vi "Read Support Script.vi"(6 "Error In":errorcluster, 8 "Support Script":path, 9 "Data In":T1={"Message"="", "Homed?"=FALSE, "NextState"=enum."Timeout", "G.Load"=0.0, "G.Position"=0.0, "Load#"=0, "[G.Loads]"=[], "[TotalLoads]"=[], "[Errors]"=[], "ZeroWait"=0, "Results"=[], "DwellWait"=FALSE, "Test Result"=FALSE, "[CondyleLoads]"=[], "[Max]"=[], "[Min]"=[], "Valid String?"=FALSE, "ScanTime"=timestamp(0 s since 1904-01-01), "ScannedString"="", "LabelDevID"=0, "MfgDate"=timestamp(0 s since 1904-01-01), "[EEPROM Cmds]"=[], "[CalData]"=[], "[A/Ds]"=[], "[A/Dmax]"=[], "[A/Dmin]"=[], "BattMax"=0.0, "BattMin"=0.0, "DwellTime"=2000, "PendingDeviceType"="", "Zero G.load"=0.0, "GAINC Value"="", "Programming Step"=enum."Load EEPROM", "Front Panel Program?"=FALSE, "Final Program?"=FALSE, "PCB Score"=100, "AssyScore"=100, "Pass/Fail #"="", "Result String"="", "Programming Mode"=enum."Initial Program", "Angle Test Step"=enum."Initialize", "Accel Values"=[], "Shutdown Counter"=0, "V1"=0, "V2"=0, "V3"=0, "V4"=0, "EEPROM Data"=[], "Counter"=0, "Page#"=0, "Timer"=timestamp(0 s since 1904-01-01), "Use Mark10?"=FALSE, "Eng-Result#"=0, "DUT Serial #"=0, "Scroll Message?"=FALSE, "Clear Message"=FALSE, "Batt Test Step "=enum."Initialize", "RXTX Window Found?"=FALSE, "Shutdown First Call?"=FALSE, "A2 Delay (msec)"=500, "Support Script"={"Script #"="", "Script Revision"="", "[OEMs]"=[], "[[DeviceTypes]]"=[], "[[DeviceTypesVals]]"=[], "[[List of Errors]]"=[], "Default GAINC"="", "[[ASICtrims]]"=[], "ID For Echo"="", "Condyle A CalFactor"=100, "Condyle B CalFactor"=100, "[OEMs Prefix]"=[], "Packet ID 18"="", "[[Force Table Load Test]]"=[], "[[Force Table AccurTest]]"=[]}, "Serial Table"={"Serial File Path"=path "", "[[Serial Lookup Table]]"=[], "Serial Device Info"=[], "Valid Serial?"=FALSE}, "Target Information"={"Target Brand"="", "Target DeviceType"="", "Target Serial#"=100, "Target Lot#"=0, "Target DevID"=0, "Target Channel"=5}, "Operator"="", "COM Port"="", "Config Path"=path "", "Tx Array"=[], "DUT Parameters"={"Channel"=0, "DeviceID"=0, "Script Rev"=0, "Month"=0, "Day"=0, "Year"=0, "Lot#"=0, "V1"=0, "V2"=0, "V3"=0, "V4"=0, "MFG"=0, "Cal FactorA 10"=0, "Cal FactorB 10  "=0, "Cal FactorA 16"=0, "Cal FactorB 16"=0, "ASICtrim"=[], "TmpChan"=0, "GAINC"="", "Brand"="", "Device"="", "Serial #"=0, "Batt310"=0, "Batt 280"=0}, "FTS Main?"=FALSE, "Loading"={"[Forces]"=[], "[Dwell]"=[], "Loading Step"=enum."Initialize Test"}, "Software Version"="", "Correction Factor"="", "Second Load Test"=FALSE, "Acc Loads"=[], "Mark10 Config"={"H2S%"=[80.0, 85.0, 90.0, 95.0, 100.0], "H2S Speed"=[12.0, 8.0, 6.0, 4.0, 2.0], "H to S"=2.0, "Home Speed"=1.0, "LoadWin"=0.0, "Load Speed"=0.0, "PID"={"Kp"=0.04, "Kd"=0.005001, "Ki"=2.9999999999999923e-05}}, "Channels"={"Transceiver Ch"=5, "Operating Ch"=5, "Start Ch"=0}, "Channel EEPROM"=[], "Load Notes"=[], "Engr Log?"=FALSE, "Time"=[], "Program Retry"=FALSE, "Operator Channel"="", "Target Channel "="", "New Data Program"=FALSE, "NFHU Pass?"=FALSE, "Cycle Number"=0, "Cal Cycle#"=0, "[Avg G.Loads] "=[], "[Avg A/Ds] "=[], "Cal Retry?"=FALSE, "[Total A/Ds]  "=[], "Cycle Num LA"=0, "LA Cycle# "=0, "Shim Num"=0, "Shim#  "=0, "Angle Test?"=FALSE} {"Mark10 Config"."PID"."Ki" min=0.0 max=200.0 format="%.6f"; "Mark10 Config"."PID"."Kd" min=0.0 max=200.0 format="%.6f"; "Mark10 Config"."PID"."Kp" min=0.0 max=200.0 format="%.6f"; "DUT Parameters"."ASICtrim" format="%02x"}) -> (0 "error out":errorcluster, 3 "Data Out":T1={"Message"="", "Homed?"=FALSE, "NextState"=enum."Timeout", "G.Load"=0.0, "G.Position"=0.0, "Load#"=0, "[G.Loads]"=[], "[TotalLoads]"=[], "[Errors]"=[], "ZeroWait"=0, "Results"=[], "DwellWait"=FALSE, "Test Result"=FALSE, "[CondyleLoads]"=[], "[Max]"=[], "[Min]"=[], "Valid String?"=FALSE, "ScanTime"=timestamp(0 s since 1904-01-01), "ScannedString"="", "LabelDevID"=0, "MfgDate"=timestamp(0 s since 1904-01-01), "[EEPROM Cmds]"=[], "[CalData]"=[], "[A/Ds]"=[], "[A/Dmax]"=[], "[A/Dmin]"=[], "BattMax"=0.0, "BattMin"=0.0, "DwellTime"=2000, "PendingDeviceType"="", "Zero G.load"=0.0, "GAINC Value"="", "Programming Step"=enum."Load EEPROM", "Front Panel Program?"=FALSE, "Final Program?"=FALSE, "PCB Score"=100, "AssyScore"=100, "Pass/Fail #"="", "Result String"="", "Programming Mode"=enum."Initial Program", "Angle Test Step"=enum."Initialize", "Accel Values"=[], "Shutdown Counter"=0, "V1"=0, "V2"=0, "V3"=0, "V4"=0, "EEPROM Data"=[], "Counter"=0, "Page#"=0, "Timer"=timestamp(0 s since 1904-01-01), "Use Mark10?"=FALSE, "Eng-Result#"=0, "DUT Serial #"=0, "Scroll Message?"=FALSE, "Clear Message"=FALSE, "Batt Test Step "=enum."Initialize", "RXTX Window Found?"=FALSE, "Shutdown First Call?"=FALSE, "A2 Delay (msec)"=500, "Support Script"={"Script #"="", "Script Revision"="", "[OEMs]"=[], "[[DeviceTypes]]"=[], "[[DeviceTypesVals]]"=[], "[[List of Errors]]"=[], "Default GAINC"="", "[[ASICtrims]]"=[], "ID For Echo"="", "Condyle A CalFactor"=100, "Condyle B CalFactor"=100, "[OEMs Prefix]"=[], "Packet ID 18"="", "[[Force Table Load Test]]"=[], "[[Force Table AccurTest]]"=[]}, "Serial Table"={"Serial File Path"=path "", "[[Serial Lookup Table]]"=[], "Serial Device Info"=[], "Valid Serial?"=FALSE}, "Target Information"={"Target Brand"="", "Target DeviceType"="", "Target Serial#"=100, "Target Lot#"=0, "Target DevID"=0, "Target Channel"=5}, "Operator"="", "COM Port"="", "Config Path"=path "", "Tx Array"=[], "DUT Parameters"={"Channel"=0, "DeviceID"=0, "Script Rev"=0, "Month"=0, "Day"=0, "Year"=0, "Lot#"=0, "V1"=0, "V2"=0, "V3"=0, "V4"=0, "MFG"=0, "Cal FactorA 10"=0, "Cal FactorB 10  "=0, "Cal FactorA 16"=0, "Cal FactorB 16"=0, "ASICtrim"=[], "TmpChan"=0, "GAINC"="", "Brand"="", "Device"="", "Serial #"=0, "Batt310"=0, "Batt 280"=0}, "FTS Main?"=FALSE, "Loading"={"[Forces]"=[], "[Dwell]"=[], "Loading Step"=enum."Initialize Test"}, "Software Version"="", "Correction Factor"="", "Second Load Test"=FALSE, "Acc Loads"=[], "Mark10 Config"={"H2S%"=[80.0, 85.0, 90.0, 95.0, 100.0], "H2S Speed"=[12.0, 8.0, 6.0, 4.0, 2.0], "H to S"=2.0, "Home Speed"=1.0, "LoadWin"=0.0, "Load Speed"=0.0, "PID"={"Kp"=0.04, "Kd"=0.005001, "Ki"=2.9999999999999923e-05}}, "Channels"={"Transceiver Ch"=5, "Operating Ch"=5, "Start Ch"=0}, "Channel EEPROM"=[], "Load Notes"=[], "Engr Log?"=FALSE, "Time"=[], "Program Retry"=FALSE, "Operator Channel"="", "Target Channel "="", "New Data Program"=FALSE, "NFHU Pass?"=FALSE, "Cycle Number"=0, "Cal Cycle#"=0, "[Avg G.Loads] "=[], "[Avg A/Ds] "=[], "Cal Retry?"=FALSE, "[Total A/Ds]  "=[], "Cycle Num LA"=0, "LA Cycle# "=0, "Shim Num"=0, "Shim#  "=0, "Angle Test?"=FALSE} {"Mark10 Config"."PID"."Ki" min=0.0 max=200.0 format="%.6f"; "Mark10 Config"."PID"."Kd" min=0.0 max=200.0 format="%.6f"; "Mark10 Config"."PID"."Kp" min=0.0 max=200.0 format="%.6f"; "DUT Parameters"."ASICtrim" format="%02x"})   [LabVIEW 2015]
uses:
  Controls/LocalVars.ctl
  Controls/Gen2 FT states.ctl
  Controls/Iniial Device Programming.ctl
  SubVI/ProgramStageControl.ctl
  Controls/Batt Cap Steps.ctl
  Controls/Support Script.ctl
  Controls/Serial Table.ctl
  Controls/Device Information.ctl
  Controls/InfoPacket.ctl
  Controls/Loading.ctl
  Controls/Load Step.ctl
  Controls/Mark10 Config.ctl
  Controls/PID parameters.ctl
  Controls/Channels.ctl
  <vilib>/Utility/NIReport.llb/NI_report.lvclass
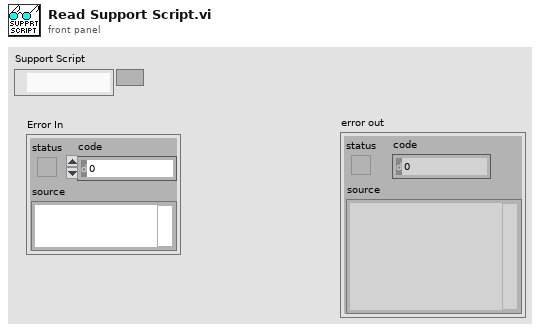
[diagram p1: front panel]
types:
  T1 = typedef "LocalVars.ctl" = cluster{"Message":string, "Homed?":bool, "NextState":T2, "G.Load":dbl, "G.Position":dbl, "Load#":i32, "[G.Loads]":dbl[], "[TotalLoads]":dbl[], "[Errors]":dbl[][], "ZeroWait":u32, "Results":dbl[], "DwellWait":bool, "Test Result":bool, "[CondyleLoads]":dbl[][], "[Max]":dbl[], "[Min]":dbl[], "Valid String?":bool, "ScanTime":timestamp, "ScannedString":string, "LabelDevID":u32, "MfgDate":timestamp, "[EEPROM Cmds]":u8[][], "[CalData]":u8[][], "[A/Ds]":dbl[][], "[A/Dmax]":dbl[], "[A/Dmin]":dbl[], "BattMax":dbl, "BattMin":dbl, "DwellTime":i32, "PendingDeviceType":string, "Zero G.load":dbl, "GAINC Value":string, "Programming Step":T3, "Front Panel Program?":bool, "Final Program?":bool, "PCB Score":i32, "AssyScore":i32, "Pass/Fail #":string, "Result String":string, "Programming Mode":T4, "Angle Test Step":enum16{"Initialize", "Get X", "Get Y", "Get Z", "Next Test"}, "Accel Values":dbl[][], "Shutdown Counter":u32, "V1":i32, "V2":i32, "V3":i32, "V4":i32, "EEPROM Data":i32[][], "Counter":i32, "Page#":i32, "Timer":timestamp, "Use Mark10?":bool, "Eng-Result#":u32, "DUT Serial #":i32, "Scroll Message?":bool, "Clear Message":bool, "Batt Test Step ":T5, "RXTX Window Found?":bool, "Shutdown First Call?":bool, "A2 Delay (msec)":i16, "Support Script":T6, "Serial Table":T7, "Target Information":T8, "Operator":string, "COM Port":string, "Config Path":path, "Tx Array":u8[], "DUT Parameters":T9, "FTS Main?":bool, "Loading":T10, "Software Version":string, "Correction Factor":string, "Second Load Test":bool, "Acc Loads":dbl[][], "Mark10 Config":T12, "Channels":T14, "Channel EEPROM":i32[][], "Load Notes":string[], "Engr Log?":bool, "Time":timestamp[], "Program Retry":bool, "Operator Channel":string, "Target Channel ":string, "New Data Program":bool, "NFHU Pass?":bool, "Cycle Number":i32, "Cal Cycle#":i32, "[Avg G.Loads] ":dbl[], "[Avg A/Ds] ":dbl[][], "Cal Retry?":bool, "[Total A/Ds]  ":dbl[][], "Cycle Num LA":i32, "LA Cycle# ":i32, "Shim Num":i32, "Shim#  ":i32, "Angle Test?":bool}
  T2 = typedef "Gen2 FT states.ctl" = enum16{"---------SETUP-------", "Initialization", "Read Support Data", "Initialize Mark-10", "Initialize Transceiver", "------UTILITIES------", "Change DUT Channel", "Find RxTx Window", "Reset Device", "Scan Channels", "Read Serial Lookup", "Shutdown Device", "ESTOP", "--------USER---------", "Timeout", "-----PROGRAM-----", "Program Device", "------MARK10--------", "Go Home", "MoveUp", "MoveDown", "Goto Load", "Goto Position", "Stop Motor", "---------TESTS--------", "Start Test", "Angle Test", "Load Test", "Load Accuracy Test", "Battery Test", "------RESULTS-------", "End Test", "Display Result", "--------EXIT--------", "Exit"}
  T3 = typedef "Iniial Device Programming.ctl" = enum16{"Load EEPROM", "Send First A1", "Send EEPROM", "Send A1", "Check EEPROM Echo", "Verify transmission", "Programming Successful", "Programming Failed"}
  T4 = typedef "ProgramStageControl.ctl" = enum16{"Initial Program", "GainC", "Scales"}
  T5 = typedef "Batt Cap Steps.ctl" = enum16{"Initialize", "Collect 2.8 Volts", "Collect 3.1 Volts", "Check Results"}
  T6 = typedef "Support Script.ctl" = cluster{"Script #":string, "Script Revision":string, "[OEMs]":string[], "[[DeviceTypes]]":string[][], "[[DeviceTypesVals]]":u16[][], "[[List of Errors]]":string[][], "Default GAINC":string, "[[ASICtrims]]":u8[][], "ID For Echo":string, "Condyle A CalFactor":i32, "Condyle B CalFactor":i32, "[OEMs Prefix]":string[], "Packet ID 18":string, "[[Force Table Load Test]]":dbl[][], "[[Force Table AccurTest]]":dbl[][]}
  T7 = typedef "Serial Table.ctl" = cluster{"Serial File Path":path, "[[Serial Lookup Table]]":string[][], "Serial Device Info":string[], "Valid Serial?":bool}
  T8 = typedef "Device Information.ctl" = cluster{"Target Brand":string, "Target DeviceType":string, "Target Serial#":i32, "Target Lot#":u32, "Target DevID":u32, "Target Channel":u8}
  T9 = typedef "InfoPacket.ctl" = cluster{"Channel":u8, "DeviceID":u32, "Script Rev":u8, "Month":u8, "Day":u8, "Year":u8, "Lot#":u32, "V1":u16, "V2":u16, "V3":u16, "V4":u16, "MFG":u8, "Cal FactorA 10":u8, "Cal FactorB 10  ":u8, "Cal FactorA 16":u8, "Cal FactorB 16":u8, "ASICtrim":u8[], "TmpChan":u8, "GAINC":string, "Brand":string, "Device":string, "Serial #":u64, "Batt310":u16, "Batt 280":u16}
  T10 = typedef "Loading.ctl" = cluster{"[Forces]":dbl[], "[Dwell]":dbl[], "Loading Step":T11}
  T11 = typedef "Load Step.ctl" = enum16{"Initialize Test", "Go Home", "Detect Dev Surface", "Wait to zero Device", "Zero Device", "Do Test", "Test Result"}
  T12 = typedef "Mark10 Config.ctl" = cluster{"H2S%":dbl[], "H2S Speed":dbl[], "H to S":dbl, "Home Speed":dbl, "LoadWin":dbl, "Load Speed":dbl, "PID":T13}
  T13 = typedef "PID parameters.ctl" = cluster{"Kp":dbl, "Kd":dbl, "Ki":dbl}
  T14 = typedef "Channels.ctl" = cluster{"Transceiver Ch":u8, "Operating Ch":u8, "Start Ch":u8}
  T15 = enum16{"Standard Report", "HTML", "Word", "Excel"}
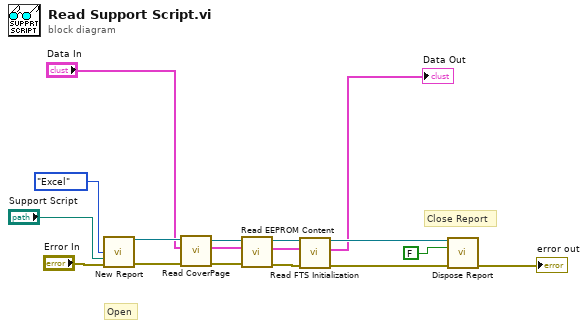
[diagram p0: block diagram]
diagram:
  # "Open"
  # "Close Report"
  n1 = call <vilib>:"New Report.vi"("report type"=T15."Excel", "template (empty)"="Support Script", "error in (no error)"="Error In") -> ("report out"=w9:refnum<class "NI_report.lvclass">, "error out"=w7:errorcluster)  [unwired: 11 in]
  n2 = call "Read CoverPage.vi"("error in (no error)"=w7, "Data In"="Data In", "NI_report in"=w9) -> ("error out"=w4:errorcluster, "Data Out"=w6:T1, "NI_report out"=w5:refnum<class "NI_report.lvclass">)  [unwired: 6 in]
  n3 = call "Read EEPROM Content.vi"("error in (no error)"=w4, "Data In"=w6, "NI_report in"=w5) -> ("error out"=w13:errorcluster, "Data Out"=w3:T1, "NI_report out"=w14:refnum<class "NI_report.lvclass">)  [unwired: 6 in]
  n4 = call "Read FTS Initialization.vi"("error in (no error)"=w13, "Data Out in"=w3, "NI_report in"=w14) -> ("error out"=w10:errorcluster, "Data Out out"=→"Data Out":T1, "report out"=w2:refnum<class "NI_report.lvclass">)  [unwired: 6 in]
  n5 = call-dynamic "Dispose Report.vi"("report in"=w2, "wait until printing completed? (T)"=FALSE, "error in (no error)"=w10) -> ("error out"=→"error out":errorcluster)  [unwired: 12 in]
